vi "DataProcess.vi"(8 "error in (no error)":errorcluster) -> (0 "error out":errorcluster)   [LabVIEW 2016]
uses:
  <vilib>/Platform/TimedLoop/XDataNode/timing_clust.ctl
  <vilib>/Platform/TimedLoop/XDataNode/nitl_modes.ctl
  <vilib>/Platform/TimedLoop/XDataNode/wakeup.ctl
  Typedef/Filter Data.ctl
  Typedef/INS Data.ctl
  <vilib>/Analysis/coordinate.llb/Wrap Angle (scalar).vi
  <vilib>/Analysis/3filter.llb/Butterworth Filter (DBL).vi
  Shared resoruces/Navigation Variables.vi
  <vilib>/platform/TimedLoop/XDataNode/XDataNode.xnode
  Shared resoruces/Shared resources RT.lvlib
  <vilib>/Analysis/NI_AALBase.lvlib
  <vilib>/Platform/TimedLoop/XDataNode/XDNodeRunTimeDep.lvlib
  <vilib>/ptbypt/NI_PtbyPt.lvlib
  <vilib>/Analysis/NI_AAL_Angle.lvlib
panel:
  in  "Curre":dbl=0.2
  out "Berro":i32
  in  "maxDiff":dbl=0.75
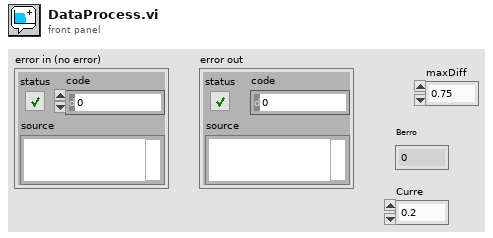
[diagram p1: front panel]
types:
  T1 = typedef "XDNodeRunTimeDep.lvlib/timing_clust.ctl" = cluster{"Expected End [f-1]":u64, "Actual End [f-1]":u64, "Finished Late? [f-1]":bool, "Expected End [i-1]":u64, "Actual End [i-1]":u64, "Finished Late? [i-1]":bool, "Expected Start [i]":u64, "Actual Start [i]":u64, "Expected Start [f]":u64, "Actual Start [f]":u64, "Source Name":string, "Structure Name":string, "Period":i64, "Deadline":i64, "Offset":i64, "Start":i64, "Priority":i32, "Timeout":i32, "Mode":T2, "Wakeup Reason":T3, "Error":errorcluster, "Source Type":string, "Secondary Source Type":string, "Global End Time":u64, "Global Start Time":u64, "Frame Duration":u64, "Iteration Duration":u64, "Assigned CPU":i32, "I/O Scan Engine Mode":u32}
  T2 = typedef "XDNodeRunTimeDep.lvlib/nitl_modes.ctl" = enum32{"No Change", "Process missed periods, maintain original phase", "Discard missed periods, maintain original phase", "Process missed periods, ignore original phase", "Discard missed periods, ignore original phase"}
  T3 = typedef "XDNodeRunTimeDep.lvlib/wakeup.ctl" = enum32{"Normal", "Aborted", "Asynchronous wakeup", "Timing source error", "Timed loop error", "Timeout"}
  T4 = typedef "Filter Data.ctl" = cluster{"Yaw":dbl, "Lat":dbl, "Long":dbl}
  T5 = typedef "INS Data.ctl" = cluster{"Yaw":sgl, "Pitch":sgl, "Roll":sgl, "Lat":dbl, "Long":dbl, "Alt":dbl, "North":dbl, "East":dbl, "Down":dbl, "PosU":dbl, "VelU":dbl}
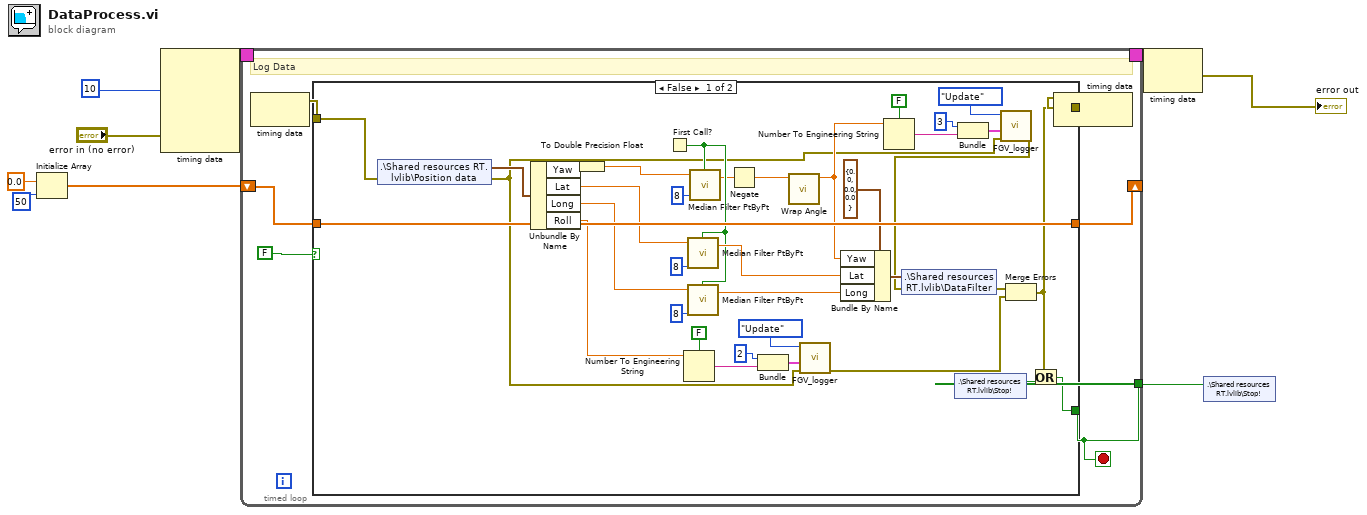
[diagram p0: block diagram]
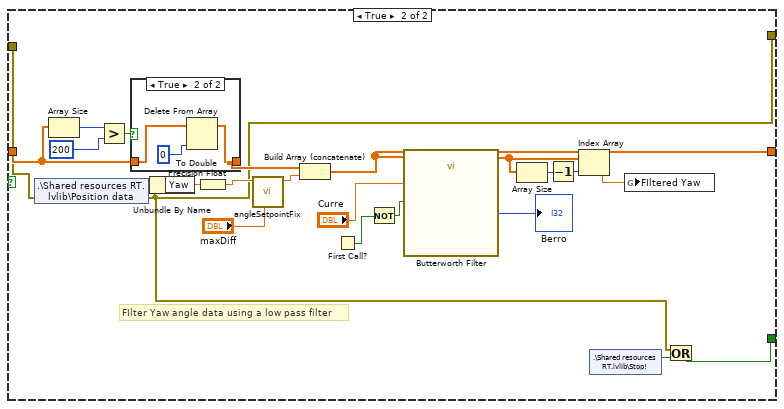
[diagram p2: hidden frame]
diagram:
  n1 = Initialize Array(0.0, 50) -> (w8:dbl[])
  n2 = node-c288(i64 10 ("Period"), "error in (no error)") -> (w5:T1)  [unwired: 3 in]
  n3 = timed-loop {
    tunnel: [w15] -> w9
    shift-right: [w13] -> _
    shift-left: w8 -> [w14]
    timing: w5 -> [_]
    timing-out: [_] -> w4
    stop <- w15 stop-if-true
    # "Log Data"
    n4 = node-c288() -> (w11:errorcluster)  [unwired: 1 in]
    n5 = case shown="False" FALSE {
      tunnel: [w48 w73] -> w15
      tunnel: w14 -> [w46 w66]
      tunnel: [w46 w58] -> w13
      tunnel: [w18 w55] -> w12
      tunnel: w11 -> [w47 w54]
      frame False {
        n6 = shared-variable ".\\Shared resources RT.lvlib\\Position data"(error in=w47) -> (w51:T5, error out=w20:errorcluster)
        n7 = Unbundle By Name(w51) -> ("Yaw"=w50:sgl, "Lat"=w39:dbl, "Long"=w38:dbl, "Roll"=w21:sgl)
        n8 = To Double Precision Float(number=w50) -> (double precision float=w45:dbl)
        n9 = First Call?() -> (First Call?: T/F=w35:bool)
        n10 = Number To Engineering String(1:FALSE ("use system decimal point (T)"), 4:w21) -> (0:w25:string)  [unwired: 2 in]
        n11 = call <vilib>:"Median Filter PtByPt.vi"("initialize"=w35, "rank"=8, "x"=w39) -> ("Filtered x"=w37:dbl)  [unwired: 1 in, 1 out]
        n12 = call <vilib>:"Median Filter PtByPt.vi"("initialize"=w35, "rank"=8, "x"=w38) -> ("Filtered x"=w36:dbl)  [unwired: 1 in, 1 out]
        n13 = call <vilib>:"Median Filter PtByPt.vi"("initialize"=w35, "rank"=8, "x"=w45) -> ("Filtered x"=w28:dbl)  [unwired: 1 in, 1 out]
        n14 = Negate(x=w28) -> (-x=w16:dbl)
        n15 = Bundle(2, w25) -> (w26:cluster{i32, string})  [unwired: 1 in]
        n16 = call-poly <vilib>:"Wrap Angle.vi"("angle in"=w16) -> ("angle out"=w27:dbl)  [unwired: 9 in, 1 out]
        n17 = call "FGV_logger.vi"("error in"=w20, 9:w26, "Command"=enum16{"Update", "Log", "Init"}."Update") -> ("error out"=w17:errorcluster)  [unwired: 8 in]
        n18 = Bundle By Name(cluster=T4 {"Yaw"=0.0, "Lat"=0.0, "Long"=0.0} ("Filter Data"), "Yaw"=w27, "Lat"=w37, "Long"=w36) -> (w42:T4)
        n19 = Number To Engineering String(1:FALSE ("use system decimal point (T)"), 4:w27) -> (0:w33:string)  [unwired: 2 in]
        n20 = shared-variable ".\\Shared resources RT.lvlib\\Stop!"() -> (w49:bool)  [unwired: 1 in, 1 out]
        n21 = Bundle(3, w33) -> (w34:cluster{i32, string})  [unwired: 1 in]
        n22 = call "FGV_logger.vi"("error in"=w20, 9:w34, "Command"=enum16{"Update", "Log", "Init"}."Update") -> ("error out"=w29:errorcluster)  [unwired: 8 in]
        n23 = shared-variable ".\\Shared resources RT.lvlib\\DataFilter"(w42, error in=w29) -> (error out=w19:errorcluster)
        n24 = Merge Errors(w19, w17) -> (w18:errorcluster)
        n25 = Or(x=w18, y=w49) -> (x .or. y?=w48:bool)
      }
      frame True {
        # "FIlter Yaw angle data using a low pass filter"
        n26 = shared-variable ".\\Shared resources RT.lvlib\\Position data"(error in=w54) -> (w69:T5, error out=w55:errorcluster)
        n27 = Array Size(array=w66) -> (size(s)=w60:i32)
        n28 = Greater?(x=w60, y=200) -> (0:w67:bool)
        n29 = case shown="True" w67 {
          tunnel: w66 -> [w75 w78]
          tunnel: [w75 w77] -> w65
          frame False {
          }
          frame True {
            n30 = Delete From Array(array=w78, index=0) -> (array with subset deleted=w77:dbl[])  [unwired: 1 in, 1 out]
          }
        }
        n31 = Unbundle By Name(w69) -> ("Yaw"=w68:sgl)
        n32 = To Double Precision Float(number=w68) -> (double precision float=w63:dbl)
        n33 = call "angleSetpointFix.vi"("maxDiff"="maxDiff", "Angle in"=w63) -> ("Angle out"=w62:dbl)  [unwired: 9 in]
        n34 = Build Array (concatenate)(w65, w62) -> (w58:dbl[])
        n35 = First Call?() -> (First Call?: T/F=w52:bool)
        n36 = Not(x=w52) -> (.not. x?=w53:bool)
        n37 = call-poly <vilib>:"Butterworth Filter.vi"("init/cont (init:F)"=w53, "low cutoff freq: fl"="Curre", "X"=w58) -> ("error"=→"Berro":i32, "Filtered X"=w61:dbl[])  [unwired: 5 in]
        n38 = Array Size(array=w61) -> (size(s)=w71:i32)
        n39 = Decrement(x=w71) -> (x-1=w70:i32)
        n40 = Index Array(array=w61, index=w70) -> (element=w72:dbl)
        n41 = shared-variable ".\\Shared resources RT.lvlib\\Stop!"() -> (w74:bool)  [unwired: 1 in, 1 out]
        n42 = global write "Navigation Variables.vi" "FIltered Yaw"(w72) -> ()
        n43 = Or(x=w55, y=w74) -> (x .or. y?=w73:bool)
      }
    }
    n44 = node-c288(w12) -> ()  [unwired: 1 out]
  }
  n45 = node-c288(w4) -> (→"error out":errorcluster)
  n46 = shared-variable ".\\Shared resources RT.lvlib\\Stop!"(w9) -> ()  [unwired: 1 in, 1 out]
